vi "Delete from Array.vi"   [LabVIEW 2016, in "JSON Value.lvclass"]
doc: "Deletes an element or subarray from a JSON array of length elements starting at index. Returns the edited array in array w/ subset deleted and the deleted element or subarray in deleted portion."
uses:
  JSON Value.lvclass
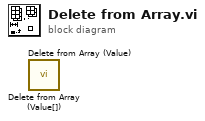
[diagram p0: block diagram]
diagram:
  n1 = call "Delete from Array (Value[]).vi"() -> ()  [unwired: 9 in, 3 out]
  n2 = call "Delete from Array (Value).vi"() -> ()  [unwired: 9 in, 3 out]
